vi "ReportHead.vi"(8 "error in (no error)":errorcluster caption="错误输入（无错误）", 11 "产品状态":string) -> (0 "error out":errorcluster caption="错误输出", 3 "report out":refnum<class "NI_report.lvclass"> caption="报表输出")   [LabVIEW 2020]
uses:
  <vilib>/Utility/NIReport.llb/NI_report.lvclass
  <vilib>/addons/_office/_exclsub.llb/font.ctl
  <vilib>/Utility/NIReport.llb/Report Type.ctl
  Global_Variable/Global.vi
  <vilib>/Utility/NIReport.llb/Append Report Text (str wrap).vi
  <vilib>/addons/_office/NI_ReportGenerationToolkit.lvlib
  <vilib>/Utility/NIReport.llb/NI_ReportGenerationCore.lvlib
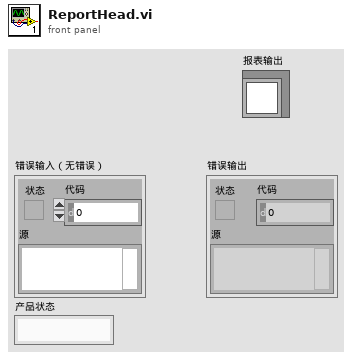
[diagram p1: front panel]
types:
  T1 = typedef "NI_ReportGenerationCore.lvlib/Report Type.ctl" = enum16{"HTML", "Word", "Excel"}
  T2 = enum16{"maximized", "minimized", "normal", "no change"}
  T3 = cluster{"操作者编号":string, "操作者姓名":string, "操作者权限":string, "联机状态":string, "产品型号":string, "产品状态":string}
  T4 = cluster{"top":dbl, "left":dbl, "right":dbl, "bottom":dbl}
  T5 = cluster{"Charset (-1)":i16, "Weight (-1)":i16, "Name":string, "Size":string}
  T6 = cluster{"Italic":enum16{"Italic Unchanged", "Italic On", "Italic Off"}, "Strike Through":enum16{"Strike Through Unchanged", "Strike Through On", "Strike Through Off"}, "Underline":enum16{"Underline Unchanged", "Underline On", "Underline Off"}, "Bold":enum16{"Bold Unchanged", "Bold On", "Bold Off"}}
  T7 = typedef "NI_ReportGenerationToolkit.lvlib/font.ctl" = cluster{"font name":string, "font size":dbl, "bold":u16, "italic":u16, "underline":u16, "strike through":u16, "font color":u32}
  T8 = cluster{"用户编号":string, "用户名":string, "用户密码(密文)":string, "用户权限":string}
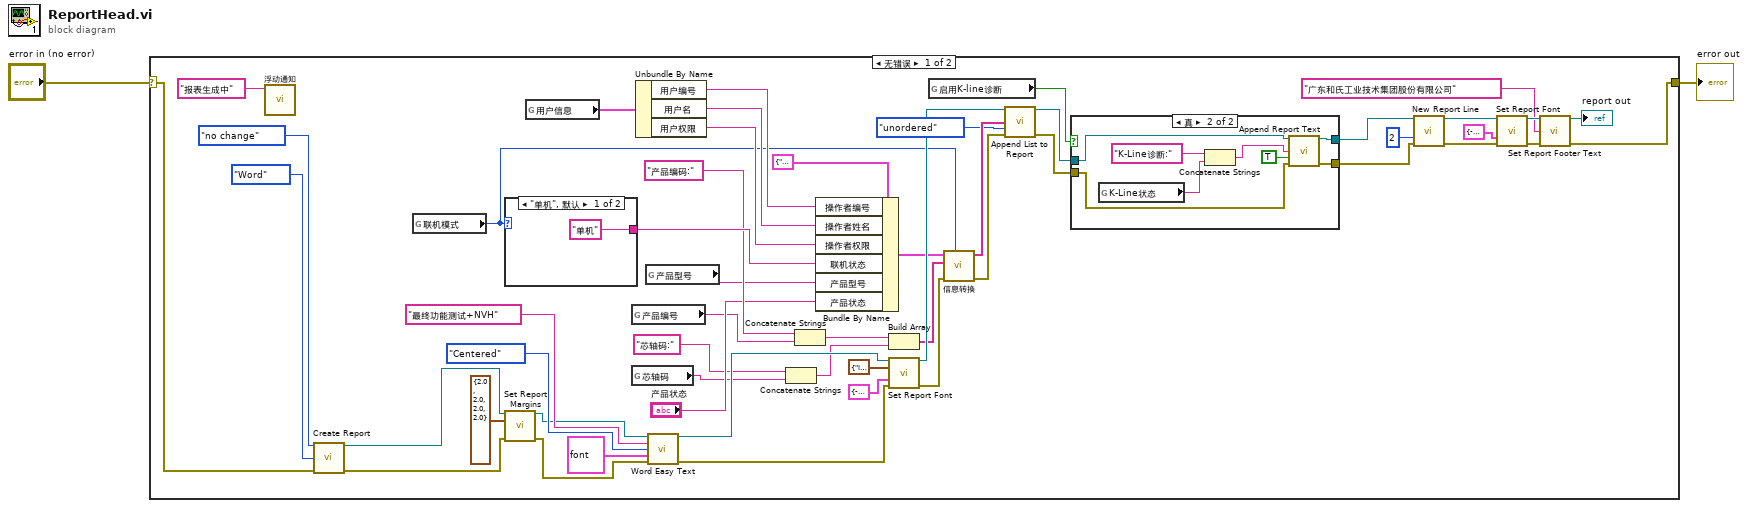
[diagram p0: block diagram]
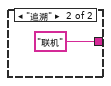
[diagram p3: hidden frame]
diagram:
  n1 = case shown="无错误" "error in (no error)" {
    selector: "error in (no error)" -> [w33 w67]
    tunnel: [w29 w67] -> w1
    frame No Error {
      n2 = call "浮动通知.vi"("通知内容"="报表生成中" ("Status")) -> ()  [unwired: 11 in]
      n3 = call <vilib>:"Create Report.vi"("window state (normal)"=T2."no change", "report type"=Report_Type."Word", "error in (no error)"=w33) -> ("report out"=w44:refnum<class "NI_report.lvclass">, "error out"=w41:errorcluster)  [unwired: 11 in]
      n4 = global read "Global.vi" "联机模式"() -> (w6:enum16{"单机", "追溯"})
      n5 = case shown="\"单机\", 默认" w6 {
        tunnel: ["单机" "联机"] -> w27
        frame "单机", Default {
        }
        frame "追溯" {
        }
      }
      n6 = call-dynamic "Set Report Margins.vi"("report in"=w44, "margins (1.00)"=T4 {"top"=2.0, "left"=2.0, "right"=2.0, "bottom"=2.0}, "error in (no error)"=w41) -> ("report out"=w43:refnum<class "NI_report.lvclass">, "error out"=w42:errorcluster)  [unwired: 10 in, 1 out]
      n7 = global read "Global.vi" "用户信息"() -> (w15:T8)
      n8 = global read "Global.vi" "产品编号"() -> (w19:string)
      n9 = global read "Global.vi" "芯轴码"() -> (w4:string)
      n10 = Unbundle By Name(w15) -> ("用户编号"=w14:string, "用户名"=w13:string, "用户权限"=w12:string)
      n11 = global read "Global.vi" "产品型号"() -> (w18:string)
      n12 = call <vilib>:"Word Easy Text.vi"("report in"=w43, "text"="最终功能测试+NVH", "alignment (left)"=enum16{"Left", "Centered", "Right", "Justify"}."Centered", "font"=T7 {"font name"="楷体", "font size"=26.0, "bold"=1, "italic"=2, "underline"=2, "strike through"=2, "font color"=16777228}, "error in (no error)"=w42) -> ("report out"=w52:refnum<class "NI_report.lvclass">, "error out"=w51:errorcluster)  [unwired: 8 in, 1 out]
      n13 = Concatenate Strings("芯轴码:", w4) -> (w3:string)
      n14 = Concatenate Strings("产品编码:", w19) -> (w23:string)
      n15 = Bundle By Name(cluster=T3 {"操作者编号"="001", "操作者姓名"="Administrator", "操作者权限"="系统管理员", "联机状态"="单机", "产品型号"="SL7202", "产品状态"=""} ("测试信息"), "操作者编号"=w14, "操作者姓名"=w13, "操作者权限"=w12, "联机状态"=w27, "产品型号"=w18, "产品状态"="产品状态") -> (w25:T3)
      n16 = Build Array(w23, w3) -> (w22:string[])
      n17 = call-dynamic "Set Report Font.vi"("report in"=w52, "text options"=T6 {"Italic"=enum."Italic Off", "Strike Through"=enum."Strike Through Unchanged", "Underline"=enum."Underline Off", "Bold"=enum."Bold Off"}, "font settings"=T5 {"Charset (-1)"=-1, "Weight (-1)"=-1, "Name"="微软雅黑 Light", "Size"="12 "}, "error in (no error)"=w51) -> ("report out"=w39:refnum<class "NI_report.lvclass">, "error out"=w32:errorcluster)  [unwired: 9 in, 1 out]
      n18 = global read "Global.vi" "启用K-line诊断"() -> (w11:bool)
      n19 = call "信息转换.vi"("联机模式"=w6, "错误输入（无错误）"=w32, "追溯码"=w22, "测试信息"=w25) -> ("错误输出"=w31:errorcluster, "信息输出"=w34:string[])  [unwired: 6 in]
      n20 = call-dynamic "Append List to Report.vi"("report in"=w39, "list elements"=w34, "list type (ordered)"=enum16{"unordered", "ordered"}."unordered", "error in (no error)"=w31) -> ("report out"=w10:refnum<class "NI_report.lvclass">, "error out"=w9:errorcluster)  [unwired: 8 in, 2 out]
      n21 = case shown="真" w11 {
        tunnel: w10 -> [w56 w61]
        tunnel: w9 -> [w55 w59]
        tunnel: [w56 w58] -> w8
        tunnel: [w55 w57] -> w7
        frame False {
        }
        frame True {
          n22 = global read "Global.vi" "K-Line状态"() -> (w63:string)
          n23 = Concatenate Strings("K-Line诊断:" ("text"), w63) -> (w62:string)
          n24 = call-poly <vilib>:"Append Report Text.vi"("report in"=w61, "text"=w62, "append on new line? (F)"=TRUE, "error in (no error)"=w59) -> ("report out"=w58:refnum<class "NI_report.lvclass">, "error out"=w57:errorcluster)  [unwired: 8 in, 2 out]
        }
      }
      n25 = call-dynamic "New Report Line.vi"("report in"=w8, "number of lines (1)"=2, "error in (no error)"=w7) -> ("report out"=w37:refnum<class "NI_report.lvclass">, "error out"=w38:errorcluster)  [unwired: 11 in]
      n26 = call-dynamic "Set Report Font.vi"("report in"=w37, "font settings"=T5 {"Charset (-1)"=-1, "Weight (-1)"=-1, "Name"="楷体", "Size"="9 "}, "error in (no error)"=w38) -> ("report out"=w48:refnum<class "NI_report.lvclass">, "error out"=w47:errorcluster)  [unwired: 10 in, 1 out]
      n27 = call-dynamic "Set Report Footer Text.vi"("report in"=w48, "center footer text"="广东和氏工业技术集团股份有限公司", "error in (no error)"=w47) -> ("report out"=→"report out":refnum<class "NI_report.lvclass">, "error out"=w29:errorcluster)  [unwired: 11 in]
    }
    frame Error {
    }
  }
  "error out" <- w1
